vi "Client TCP Request Download.vi"(8 "error in (no error)":errorcluster, 10 "File URL (empty)":path, 11 "Client (\"\": localhost)":string) -> (0 "error out":errorcluster)   [LabVIEW 2011]
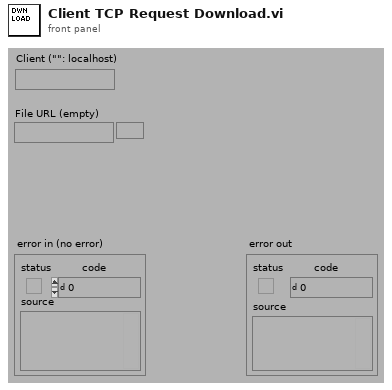
[diagram p1: front panel]
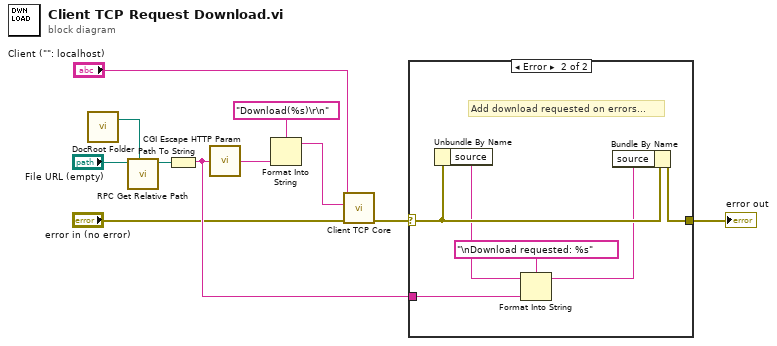
[diagram p0: block diagram]
diagram:
  n1 = call "DocRoot Folder.vi"() -> ("DocumentRoot Folder"=w9:path)  [unwired: 3 in]
  n2 = call "RPC Get Relative Path.vi"("Base Path (empty)"=w9, "Absolute Path (empty)"="File URL (empty)") -> ("Path Relative to Base"=w8:path)  [unwired: 3 out]
  n3 = Path To String(path=w8) -> (string=w3:string)
  n4 = call "CGI Escape HTTP Param.vi"("string"=w3) -> ("url-encoded string"=w4:string)
  n5 = Format Into String(format string="Download(%s)\r\n", w4) -> (resulting string=w7:string)  [unwired: 2 in, 1 out]
  n6 = call "Client TCP Core.vi"("error in (no error)"="error in (no error)", "Command(Params) (\"\")"=w7, "Client (\"\": localhost)"="Client (\"\": localhost)") -> ("error out"=w1:errorcluster)  [unwired: 8 out]
  n7 = case shown="Error" w1 {
    selector: w1 -> [w12 w16]
    tunnel: [w12 w15] -> w5
    tunnel: w3 -> [_ w17]
    frame No Error {
    }
    frame Error {
      # "Add download requested on errors..."
      n8 = Unbundle By Name(w16) -> ("source"=w14:string)
      n9 = Format Into String(format string="\nDownload requested: %s", initial string=w14, w17) -> (resulting string=w13:string)  [unwired: 1 in, 1 out]
      n10 = Bundle By Name(cluster=w16, "source"=w13) -> (w15:errorcluster)
    }
  }
  "error out" <- w5
